vi "VI Server_Generate Selected Controls Cluster.vi"(8 "error in (no error)":errorcluster, 9 "Selected Control Labels":string[](array[string]), 11 "VI Server Cluster":T1) -> (0 "error out":errorcluster, 3 "VI Server Cluster.OUT":T1)   [LabVIEW 2020, in "VI Server Toolkit LV2013.lvlib"]
doc: "Generates <B>VI Server Cluster</B> containing targeted/called VI reference, array of controls/indicators labels and corresponding array of these controls generic references.\n\nThe labels and reference arrays are <B>ONLY</B> for controls listed in <B>Selected Control Labels</B> input.\nGeneric reference is referred to as reference indifferent to the control data type."
uses:
  VI Server Toolkit LV2013.lvlib
  VI Server_TypeDefs/VI Server_RefsCluster.ctl
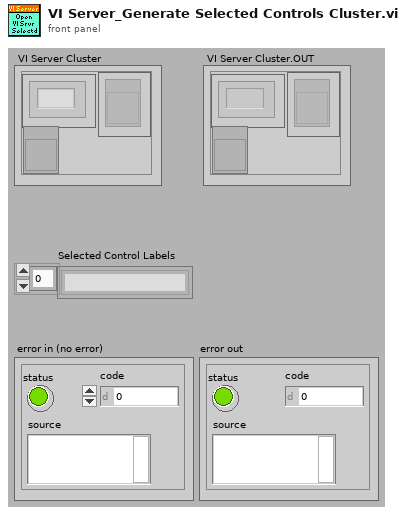
[diagram p1: front panel]
types:
  T1 = typedef "VI Server_RefsCluster.ctl" = cluster{"Labels":string[], "Refs":refnum<vi>[], "VI Ref":refnum<vi>}
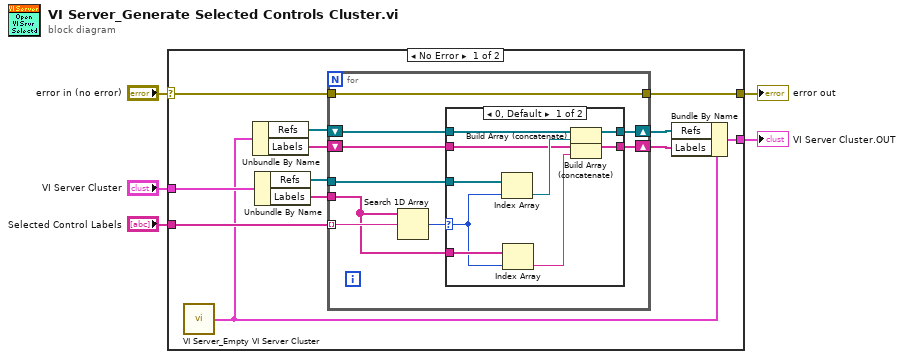
[diagram p0: block diagram]
diagram:
  n1 = case shown="No Error" "error in (no error)" {
    selector: "error in (no error)" -> [w16 w38]
    tunnel: "VI Server Cluster" -> [w17 _]
    tunnel: [w13 w38] -> w4
    tunnel: "Selected Control Labels" -> [w12 _]
    tunnel: [w11 _] -> w2
    frame No Error {
      n2 = call "VI Server_Empty VI Server Cluster.vi"() -> ("VI Server Cluster"=w6:T1)  [unwired: 7 in]
      n3 = Unbundle By Name(w6) -> ("Refs"=w10:refnum<vi>[], "Labels"=w9:string[])
      n4 = Unbundle By Name(w17) -> ("Refs"=w15:refnum<vi>[], "Labels"=w14:string[])
      n5 = for {
        tunnel: w16 -> [w26]
        tunnel: [w26] -> w13
        tunnel: w12 -> [w23] mode=indexing
        tunnel: w15 -> [w24]
        tunnel: w14 -> [w18]
        shift-right: [w19] -> w7
        shift-left: w9 -> [w20]
        shift-right: [w21] -> w8
        shift-left: w10 -> [w22]
        n6 = Search 1D Array(1D array=w18, element=w23) -> (index of element=w25:i32)  [unwired: 1 out]
        n7 = case shown="0, Default" w25 {
          selector: w25 -> [w27 _]
          tunnel: w24 -> [w35 _]
          tunnel: w22 -> [w33 w37]
          tunnel: [w32 w37] -> w21
          tunnel: w20 -> [w30 w36]
          tunnel: [w28 w36] -> w19
          tunnel: w18 -> [w34 _]
          frame 0, Default {
            n8 = Index Array(array=w35, index=w27) -> (element=w31:refnum<vi>)
            n9 = Index Array(array=w34, index=w27) -> (element=w29:string)
            n10 = Build Array (concatenate)(w33, w31) -> (w32:refnum<vi>[])
            n11 = Build Array (concatenate)(w30, w29) -> (w28:string[])
          }
          frame -1 {
          }
        }
      }
      n12 = Bundle By Name(cluster=w6, "Refs"=w8, "Labels"=w7) -> (w11:T1)
    }
    frame Error {
    }
  }
  "error out" <- w4
  "VI Server Cluster.OUT" <- w2
